vi "Configure Demodulation.vi"(0 "VISA resource name":refnum<visa-resource-name>, 1 "FM Demodulation Squelch (0)":i32, 2 "Enable Demodulation View (T: Enable)":bool=TRUE, 3 "Enable Speaker (T: Enable)":bool=TRUE, 5 "Demodulation Type (0: Off)":u16(ring) items=["Off", "FM", "AM"], 7 "FM Deviation (100000 Hz)":dbl=100000.0, 9 "FM Demodulation Time (0.5 s)":dbl=0.5, 11 "error in (no error)":errorcluster) -> (4 "VISA resource name out":refnum<visa-resource-name>, 15 "error out":errorcluster)   [LabVIEW 2014, in "Agilent ESA PSA Series.lvlib"]
doc: "Configures Demodulation.\n\n<B>Note:</B>\n\nOnly valid for ESA Series"
uses:
  Agilent ESA PSA Series.lvlib
panel:
  # "FM Demodulation Settings"
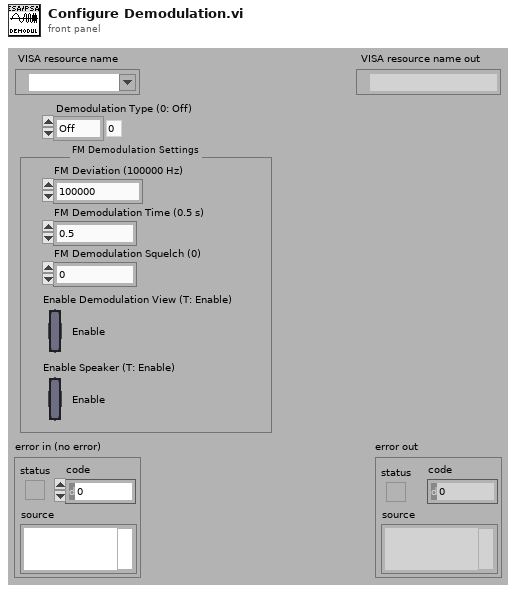
[diagram p1: front panel]
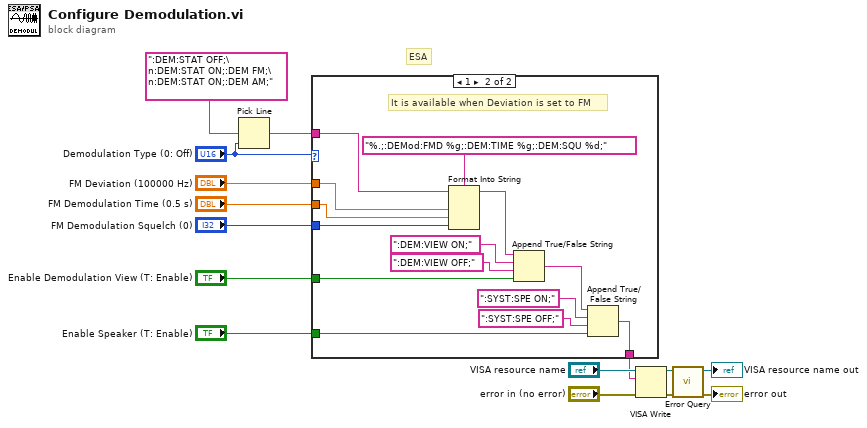
[diagram p0: block diagram]
diagram:
  # "ESA"
  n1 = Pick Line(multi-line string=":DEM:STAT OFF;\n:DEM:STAT ON;:DEM FM;\n:DEM:STAT ON;:DEM AM;", line index="Demodulation Type (0: Off)") -> (output string=w7:string)  [unwired: 1 in]
  n2 = case shown="1" "Demodulation Type (0: Off)" {
    tunnel: "FM Deviation (100000 Hz)" -> [_ w30]
    tunnel: w7 -> [w16 w28]
    tunnel: "FM Demodulation Time (0.5 s)" -> [_ w27]
    tunnel: "FM Demodulation Squelch (0)" -> [_ w26]
    tunnel: [w16 w19] -> w4
    tunnel: "Enable Demodulation View (T: Enable)" -> [_ w18]
    tunnel: "Enable Speaker (T: Enable)" -> [_ w17]
    frame 0, Default {
    }
    frame 1 {
      # "It is available when Deviation is set to FM"
      n3 = Format Into String(format string="%.;:DEMod:FMD %g;:DEM:TIME %g;:DEM:SQU %d;", initial string=w28, w30, w27, w26) -> (resulting string=w23:string)  [unwired: 1 in, 1 out]
      n4 = Append True/False String(1:w18, 2:":DEM:VIEW OFF;" ("false string"), 3:":DEM:VIEW ON;" ("false string"), 4:w23) -> (0:w22:string)
      n5 = Append True/False String(1:w17, 2:":SYST:SPE OFF;" ("true string"), 3:":SYST:SPE ON;" ("true string"), 4:w22) -> (0:w19:string)
    }
  }
  n6 = VISA Write(VISA resource name="VISA resource name", write buffer=w4, error in (no error)="error in (no error)") -> (VISA resource name out=w13:refnum<visa-resource-name>, error out=w11:errorcluster)  [unwired: 1 out]
  n7 = call "Error Query.vi"("error in (no error)"=w11, "VISA resource name"=w13) -> ("error out"=→"error out":errorcluster, "VISA resource name out"=→"VISA resource name out":refnum<visa-resource-name>)  [unwired: 6 in, 2 out]
